vi "close_cam_topLvl_v02.vi"(8 "error in (no error)":errorcluster, 11 "cam info in":T1={"camera type"=enum."Qcam", "cam handle"=0, "data handle"=0, "cam size"=[]}) -> (0 "error out":errorcluster)   [LabVIEW 2015]
uses:
  controls/cam_info.ctl
  controls/cam_type-v02.ctl
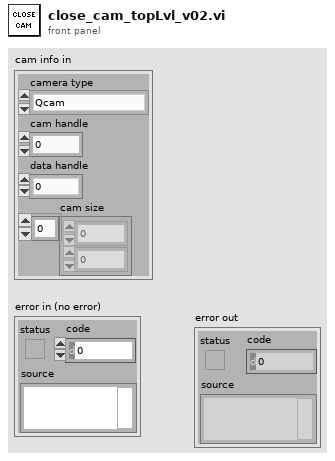
[diagram p1: front panel]
types:
  T1 = typedef "cam_info.ctl" = cluster{"camera type":T2, "cam handle":u32, "data handle":u32, "cam size":i32[]}
  T2 = typedef "cam_type-v02.ctl" = enum16{"HamamatsuORCA05G", "Qcam", "optiMOS"}
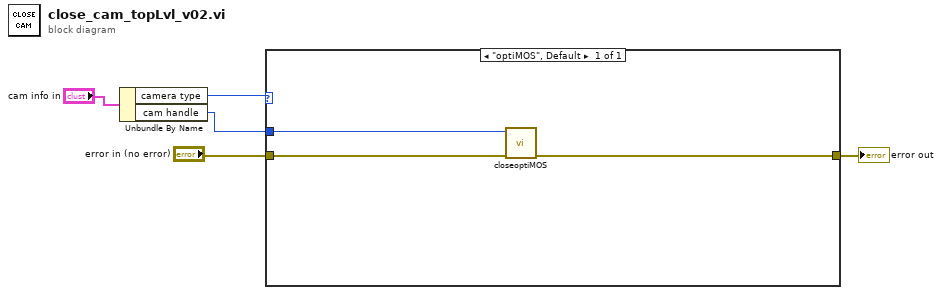
[diagram p0: block diagram]
diagram:
  n1 = Unbundle By Name("cam info in") -> ("camera type"=w5:T2, "cam handle"=w3:u32)
  n2 = case shown="\"optiMOS\", Default" w5 {
    tunnel: w3 -> [w8]
    tunnel: "error in (no error)" -> [w7]
    tunnel: [w6] -> w1
    frame "optiMOS", Default {
      n3 = call "closeoptiMOS.vi"("error in (no error)"=w7, "Camera Handle"=w8) -> ("error out"=w6:errorcluster)  [unwired: 7 in]
    }
  }
  "error out" <- w1
